vi "Data Split when each number.vi"() -> ()   [LabVIEW 2023]
panel:
  in  "floor(x/y)":i32
  in  "current Data path":path
  in  "error in":errorcluster
  in  "previous data REF":refnum<file>
  in  "split at each number":i32=3000
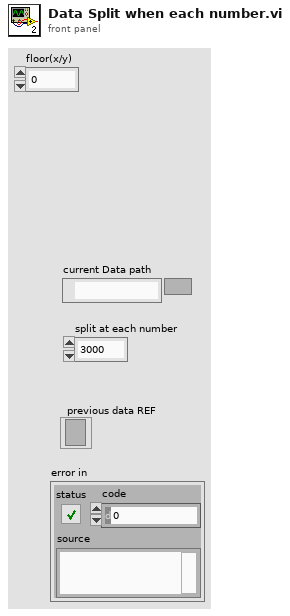
[diagram p1: front panel]
types:
  T1 = enum16{"open", "replace", "create", "open or create", "replace or create", "replace or create with confirmation"}
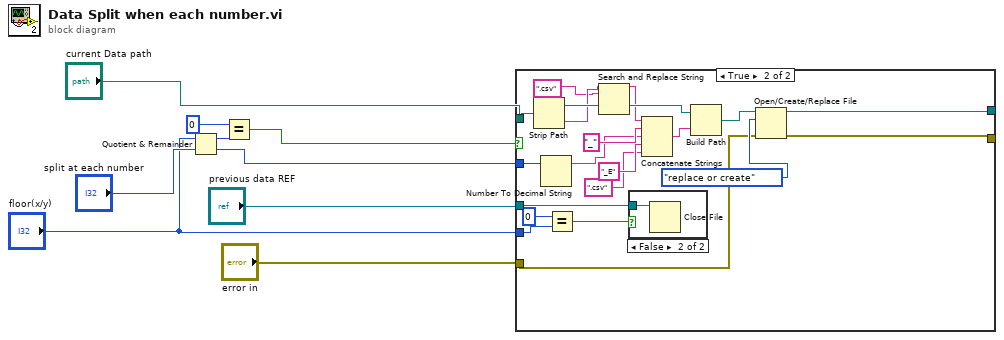
[diagram p0: block diagram]
diagram:
  n1 = Quotient & Remainder(x="floor(x/y)", y="split at each number") -> (x-y*floor(x/y)=w9:i32, floor(x/y)=w6:i32)
  n2 = Equal?(x=0, y=w9) -> (x = y?=w7:bool)
  n3 = case shown="True" w7 {
    tunnel: "current Data path" -> [_ w25]
    tunnel: w6 -> [_ w27]
    tunnel: [w10 w22] -> _
    tunnel: "error in" -> [w11 w21]
    tunnel: [w11 w20] -> _
    tunnel: "previous data REF" -> [w10 w19]
    tunnel: "floor(x/y)" -> [_ w17]
    frame False {
    }
    frame True {
      n4 = Strip Path(path=w25) -> (stripped path=w31:path, name=w13:string)
      n5 = Number To Decimal String(number=w27) -> (decimal integer string=w26:string)  [unwired: 1 in]
      n6 = Equal?(x=0, y=w17) -> (x = y?=w15:bool)
      n7 = Search and Replace String(input string=w13, search string=".csv") -> (result string=w14:string)  [unwired: 6 in, 3 out]
      n8 = case shown="False" w15 {
        tunnel: w19 -> [_ w32]
        frame True {
        }
        frame False {
          n9 = Close File(refnum=w32) -> ()  [unwired: 1 in, 2 out]
        }
      }
      n10 = Concatenate Strings(w14, "_" ("string"), w26, "_E" ("string"), ".csv" ("string")) -> (w30:string)
      n11 = Build Path(base path=w31, name or relative path=w30) -> (appended path=w23:path)
      n12 = Open/Create/Replace File(file path (use dialog)=w23, error in=w21, operation (0:open)=T1."replace or create") -> (refnum out=w22:refnum<file>, error out=w20:errorcluster)  [unwired: 3 in, 1 out]
    }
  }
